vi "UDT_programControlModule_PreRunCTRL.vi"() -> (3 "Unit Test Framework Results":T1)   [LabVIEW 2017]
doc: "Use this template to create a user-defined test VI. Define your test requirements and wire the results to the <b>Result (Test)</b> control. Do not modify the <b>Unit Test Framework Results</b> indicator."
uses:
  <vilib>/utf/common/utf_test_result_troll.ctl
  <vilib>/utf/common/utf_test_result.ctl
  <vilib>/utf/common/utf_test_result_failure.ctl
  <vilib>/utf/common/utf_test_comparison_operators.ctl
  <vilib>/utf/common/utf_vi_tag.ctl
  RT/programControl/Queue/TypeDefs/queueFGVState.ctl
  RT/programControl/Queue/TypeDefs/message.ctl
  RT/programControl/StartUEFGV/TypeDefs/UEFGVcontrol.ctl
  <vilib>/Control Software Solutions Ltd/UTF Helper/SubVIs/UTF Variant Equals.vi
  <vilib>/Control Software Solutions Ltd/UTF Helper/Unit Test Helper.lvlib
  RT/programControl/programControl.lvlib
  <vilib>/utf/NI_UnitTestFramework.lvlib
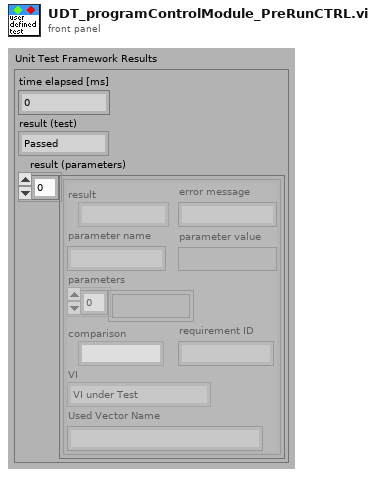
[diagram p1: front panel]
types:
  T1 = typedef "NI_UnitTestFramework.lvlib/utf_test_result_troll.ctl" = cluster{"time elapsed [ms]":u32, "result (test)":T2, "result (parameters)":T3[]}
  T2 = typedef "NI_UnitTestFramework.lvlib/utf_test_result.ctl" = enum16{"Passed", "Failed", "Error", "Skipped", "Not Processed"}
  T3 = typedef "NI_UnitTestFramework.lvlib/utf_test_result_failure.ctl" = cluster{"result":T2, "error message":string, "parameter name":string, "parameter value":variant, "parameters":variant[], "comparison":T4, "requirement ID":string, "VI":T5, "Used Vector Name":string}
  T4 = typedef "NI_UnitTestFramework.lvlib/utf_test_comparison_operators.ctl" = enum16{"=", "!=", ">", ">=", "<", "<=", "range", "symmetric tolerance", "asymmetric tolerance", "string contains", "string not contain", "array size", "string length", "array range", "by element", "array range (limit array)", "user-defined", "array contains", "array not contain", "vector length", "= (elm)", "!= (elm)", "= (case insensitive)", "!= (case insensitive)"}
  T5 = typedef "NI_UnitTestFramework.lvlib/utf_vi_tag.ctl" = enum16{"Setup VI", "VI under Test", "Teardown VI"}
  T6 = typedef "UEFGVcontrol.ctl" = enum16{"Create", "Get", "Destroy"}
  T7 = typedef "programControl.lvlib/queueFGVState.ctl" = enum16{"obtain", "enqueue (low priority)", "enqueue (high priority)", "dequeue", "release"}
  T8 = typedef "programControl.lvlib/message.ctl" = cluster{"calling module":string, "message":string, "Data":variant}
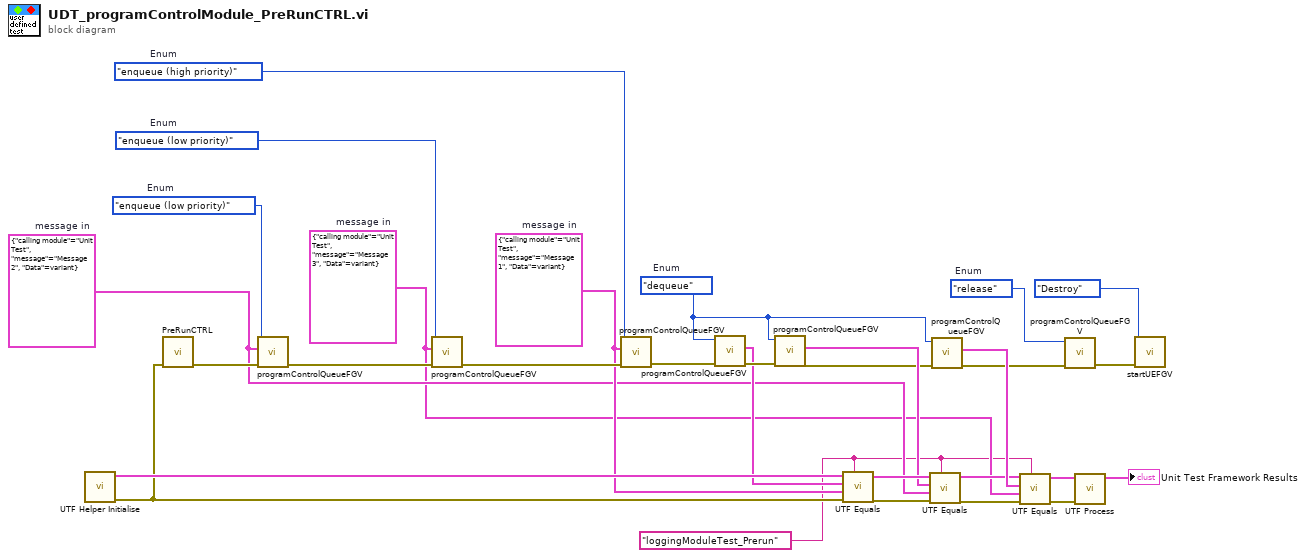
[diagram p0: block diagram]
diagram:
  w4 = "loggingModuleTest_Prerun"
  w5 = queueFGVState."release"  # Enum
  w13 = queueFGVState."dequeue"  # Enum
  w22 = T8 {"calling module"="Unit Test", "message"="Message 1", "Data"=variant}  # message in
  w9 = T8 {"calling module"="Unit Test", "message"="Message 3", "Data"=variant}  # message in
  w15 = T8 {"calling module"="Unit Test", "message"="Message 2", "Data"=variant}  # message in
  w26 = queueFGVState."enqueue (high priority)"  # Enum
  w28 = queueFGVState."enqueue (low priority)"  # Enum
  w29 = queueFGVState."enqueue (low priority)"  # Enum
  n1 = call <vilib>:"UTF Helper Initialise.vi"() -> ("error out"=w23:errorcluster, "results array"=w24:T3[])  [unwired: 10 in]
  n2 = call "PreRunCTRL.vi"("error in (no error)"=w23) -> ("error out"=w30:errorcluster)  [unwired: 10 in]
  n3 = call "programControlQueueFGV.vi"("error in (no error)"=w30, "message in"=w15, "Enum"=w29) -> ("error out"=w27:errorcluster)  [unwired: 7 in, 1 out]
  n4 = call "programControlQueueFGV.vi"("error in (no error)"=w27, "message in"=w9, "Enum"=w28) -> ("error out"=w25:errorcluster)  [unwired: 7 in, 1 out]
  n5 = call "programControlQueueFGV.vi"("error in (no error)"=w25, "message in"=w22, "Enum"=w26) -> ("error out"=w21:errorcluster)  [unwired: 7 in, 1 out]
  n6 = call "programControlQueueFGV.vi"("error in (no error)"=w21, "Enum"=w13) -> ("error out"=w18:errorcluster, "message out"=w17:T8)  [unwired: 8 in]
  n7 = call "programControlQueueFGV.vi"("error in (no error)"=w18, "Enum"=w13) -> ("error out"=w14:errorcluster, "message out"=w16:T8)  [unwired: 8 in]
  n8 = call-poly <vilib>:"UTF Equals.vi"("Parameter Name"=w4, "error in (no error)"=w23, "Test Value"=w22, "Input"=w17, "Input Results"=w24) -> ("error out"=w20:errorcluster, "Output Results"=w19:T3[])  [unwired: 5 in]
  n9 = call-poly <vilib>:"UTF Equals.vi"("Parameter Name"=w4, "error in (no error)"=w20, "Test Value"=w15, "Input"=w16, "Input Results"=w19) -> ("error out"=w10:errorcluster, "Output Results"=w11:T3[])  [unwired: 5 in]
  n10 = call "programControlQueueFGV.vi"("error in (no error)"=w14, "Enum"=w13) -> ("error out"=w6:errorcluster, "message out"=w12:T8)  [unwired: 8 in]
  n11 = call-poly <vilib>:"UTF Equals.vi"("Parameter Name"=w4, "error in (no error)"=w10, "Test Value"=w9, "Input"=w12, "Input Results"=w11) -> ("error out"=w7:errorcluster, "Output Results"=w8:T3[])  [unwired: 5 in]
  n12 = call "programControlQueueFGV.vi"("error in (no error)"=w6, "Enum"=w5) -> ("error out"=w2:errorcluster)  [unwired: 8 in, 1 out]
  n13 = call <vilib>:"UTF Process.vi"("error in (no error)"=w7, "results array"=w8) -> ("Unit Test Framework Results"=→"Unit Test Framework Results":T1)  [unwired: 9 in]
  n14 = call "startUEFGV.vi"("error in (no error)"=w2, "Enum"=UEFGVcontrol."Destroy") -> ()  [unwired: 8 in, 2 out]
